vi "Build Result Table.vi"(1 "precision (1)":i16=1 min=0, 2 "unit label":string, 3 "band power":dbl[](array[numeric]) format="%.2f", 4 "nominal frequencies (string)":string[](array[string])) -> (0 "result table":string[][](table))   [LabVIEW 2017]
doc: "Generates a table based on the results of a fractional-octave analysis. The first column of the table contains the nominal frequencies. The second column contains the band power with the appropriate unit label."
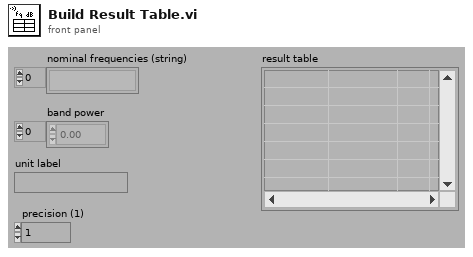
[diagram p1: front panel]
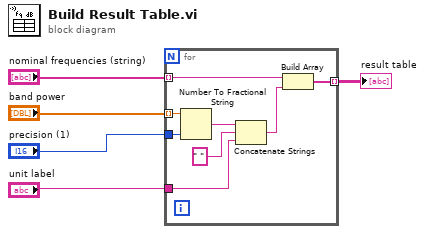
[diagram p0: block diagram]
diagram:
  n1 = for {
    tunnel: "band power" -> [w13] mode=indexing
    tunnel: "precision (1)" -> [w12]
    tunnel: "nominal frequencies (string)" -> [w11] mode=indexing
    tunnel: [w9] -> w2 mode=indexing
    tunnel: "unit label" -> [w6]
    n2 = Number To Fractional String(number=w13, precision (6)=w12) -> (F-format string=w10:string)  [unwired: 2 in]
    n3 = Concatenate Strings(w10, " ", w6) -> (w8:string)
    n4 = Build Array(w11, w8) -> (w9:string[])
  }
  "result table" <- w2
